vi "Ammeter Test Communications (648X).vi"(8 "error in (no error)":errorcluster, 11 "VISA resource name in":refnum<visa-resource-name>) -> (0 "error out":errorcluster, 3 "VISA resource name out":refnum<visa-resource-name>)   [LabVIEW 2016, in "Hall Effect Library.lvlib"]
uses:
  Hall Effect Library.lvlib
  <instrlib>/Keithley 648X/Keithley 648X.lvlib
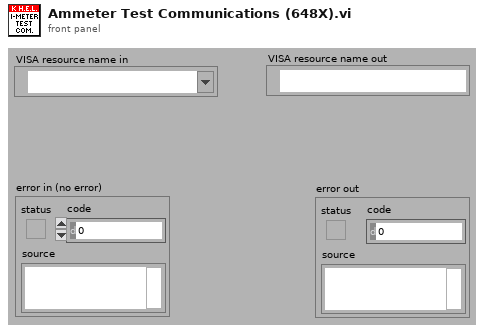
[diagram p1: front panel]
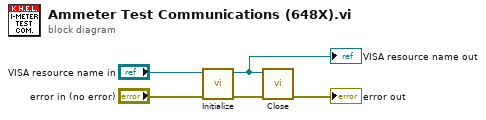
[diagram p0: block diagram]
diagram:
  n1 = call <instrlib>:"Initialize.vi"("error in (no error)"="error in (no error)", "VISA resource name"="VISA resource name in") -> ("error out"=w5:errorcluster, "VISA resource name out"=w1:refnum<visa-resource-name>)  [unwired: 3 in, 5 out]
  "VISA resource name out" <- w1
  n2 = call <instrlib>:"Close.vi"("error in (no error)"=w5, "VISA resource name"=w1) -> ("error out"=→"error out":errorcluster)  [unwired: 9 out]
